vi "Update experiment path indicator.vi"(8 "error in (no error)":errorcluster, 11 "created path":path) -> (0 "error out":errorcluster, 3 "created path (dup)":path)   [LabVIEW 2013]
uses:
  Global Variables/gl_UI Ctrl Refs.vi
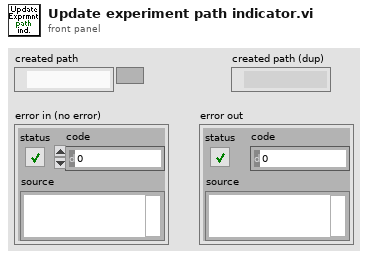
[diagram p1: front panel]
types:
  T1 = typedef "UI ctrl refs cluster.ctl" = cluster{"Top level VI path":path, "Top level VI ref":refnum<vi>, "User menu ref":refnum<k9>, "Sub Panel control":refnum<vi>, "Imaging Param Tab":refnum<vi>, "Occurrence-Start drivers":refnum<k4>, "Occurrence-Speed logging initialised":refnum<k4>, "Occurrence-XYZ stage initialised":refnum<k4>, "Exit button":refnum<vi>, "Status ind":refnum<vi>, "Return to Origin":refnum<vi>, "Speed Logging":refnum<vi>, "Time Lapse":refnum<vi>, "Live Imaging":refnum<vi>, "AOL Z Stack":refnum<vi>, "Motor Z Stack":refnum<vi>, "Funct Acq button":refnum<vi>, "Hard Shutter":refnum<vi>, "Virtual Shutter":refnum<vi>, "Laser Power":refnum<vi>, "AOL Mode":refnum<vi>, "Frame Size":refnum<vi>, "Field of View":refnum<vi>, "Dwell Time":refnum<vi>, "Zoom":refnum<vi>, "AOL Z":refnum<vi>, "Objective":refnum<vi>, "Axis":refnum<vi>, "Paths & Names":refnum<vi>, "Experiment folder path (ind.)":refnum<vi>, "Last State (Ind.)":refnum<vi>, "Laser wavelength ind (nm)":refnum<vi>, "Averages":refnum<vi>, "Angle (degrees)":refnum<vi>, "X centre":refnum<vi>, "Y centre":refnum<vi>, "Plane Mode":refnum<vi>, "# Planes":refnum<vi>, "Z Start":refnum<vi>, "Z Stop":refnum<vi>, "Z Step":refnum<vi>, "PMT 1":refnum<vi>, "PMT 2":refnum<vi>, "Stage XYZ Position":refnum<vi>, "Pockels@Z Start":refnum<vi>, "Pockels@Z Stop":refnum<vi>, "Obtain Z Start":refnum<vi>, "Obtain Z Stop":refnum<vi>, "Live stim.trig.period":refnum<vi>, "Live stim.trig.enable":refnum<vi>, "Funct. Acq. Pockels Modulation":refnum<vi>, "Enable Video Recording":refnum<vi>, "Video Record-Live Imaging":refnum<vi>, "Video Record-Funct acq":refnum<vi>, "AOL Z-stack Chirps Ready (ind)":refnum<vi>, "Center freq ind (nm)":refnum<vi>, "Logging queue (ind)":refnum<vi>, "Back aperture power (ind.)":refnum<vi>, "Power after objective (ind.)":refnum<vi>, "Switch user":refnum<vi>}
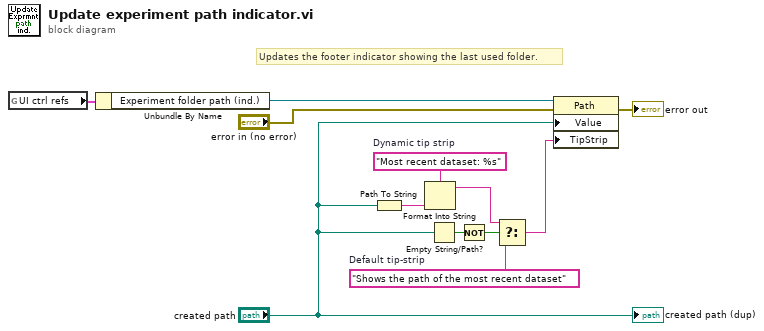
[diagram p0: block diagram]
diagram:
  w1 = "Shows the path of the most recent dataset"  # Default tip-strip
  w8 = "Most recent dataset: %s"  # Dynamic tip strip
  # "Updates the footer indicator showing the last used folder."
  n1 = global read "gl_UI Ctrl Refs.vi" "UI ctrl refs"() -> (w12:T1)
  n2 = Unbundle By Name(w12) -> ("Experiment folder path (ind.)"=w9:refnum<vi>)
  n3 = Path To String(path="created path") -> (string=w7:string)
  n4 = Format Into String(format string=w8, w7) -> (resulting string=w3:string)  [unwired: 2 in, 1 out]
  n5 = Empty String/Path?(string/path="created path") -> (empty?=w5:bool)
  n6 = Not(x=w5) -> (.not. x?=w4:bool)
  n7 = Select(t=w3, s=w4, f=w1) -> (s? t:f=w2:string)
  n8 = property on="Property Node" class="Path"(reference=w9, error in="error in (no error)", "Value"="created path", "TipStrip"=w2) -> (error out=→"error out":errorcluster)  [unwired: 1 out]
  "created path (dup)" <- "created path"
